vi "gui for machine parameters.vi"() -> ()   [LabVIEW 2025]
uses:
  control modification.ctl
  Control 5.ctl
  horizontal slide control.ctl
  counterweight load control.ctl
  time control.ctl
  <vilib>/picture/picture.llb/imagedata.ctl
  Control 6.ctl
  <vilib>/picture/picture.llb/Draw True-Color Pixmap.vi
panel:
  in  "stop 3":bool
  in  "dimension size":i32
  in  "Tank 3":T1 scale=0.0..100.0
  in  "Tank 2":T1 scale=0.0..100.0
  in  "Table 3":T2
  in  "?":bool
  in  "?":bool
  in  "?":bool
  in  "?":bool
  in  "?":bool
  in  "?":bool
  in  "?":bool
  in  "?":bool
  out "image data 2":T3
  in  "path to PNG file 2":path=path "C:/Dhanush/Dhanush/Vehicle articulated (1).PNG"
  in  "Rotation Angle (degree) 2":dbl(knob) scale=-180.0..180.0
  in  "Scale 2":dbl(slide)=1.0 scale=0.1..10.0
  in  "stop 2":bool
  out "?":picture
  out "?":T4
  out "?":T5 scale=0.0..6.0
  out "?":T5 scale=0.0..6.0
  out "image data":T3
  in  "path to PNG file":path=path "C:/Dhanush/Dhanush/Vehicle articulated (1).PNG"
  in  "Rotation Angle (degree)":dbl(knob) scale=-180.0..180.0
  in  "Scale":dbl(slide)=1.0 scale=0.1..10.0
  in  "stop":bool
  out "?":picture
  out "?":T4
  out "?":T6 scale=0.0..100.0
  in  "Table 2":T2
  in  "?":T7
  # "No of Cycles"
  # "Holding Time"
  # "Y axis Angle"
  # "Pressure"
  # "Automatic Mode Parameter Settings"
  # "Y axis"
  # "X axis"
  # "Cycle"
  # "Settings"
  # "%"
  # "Overall Progress Bar"
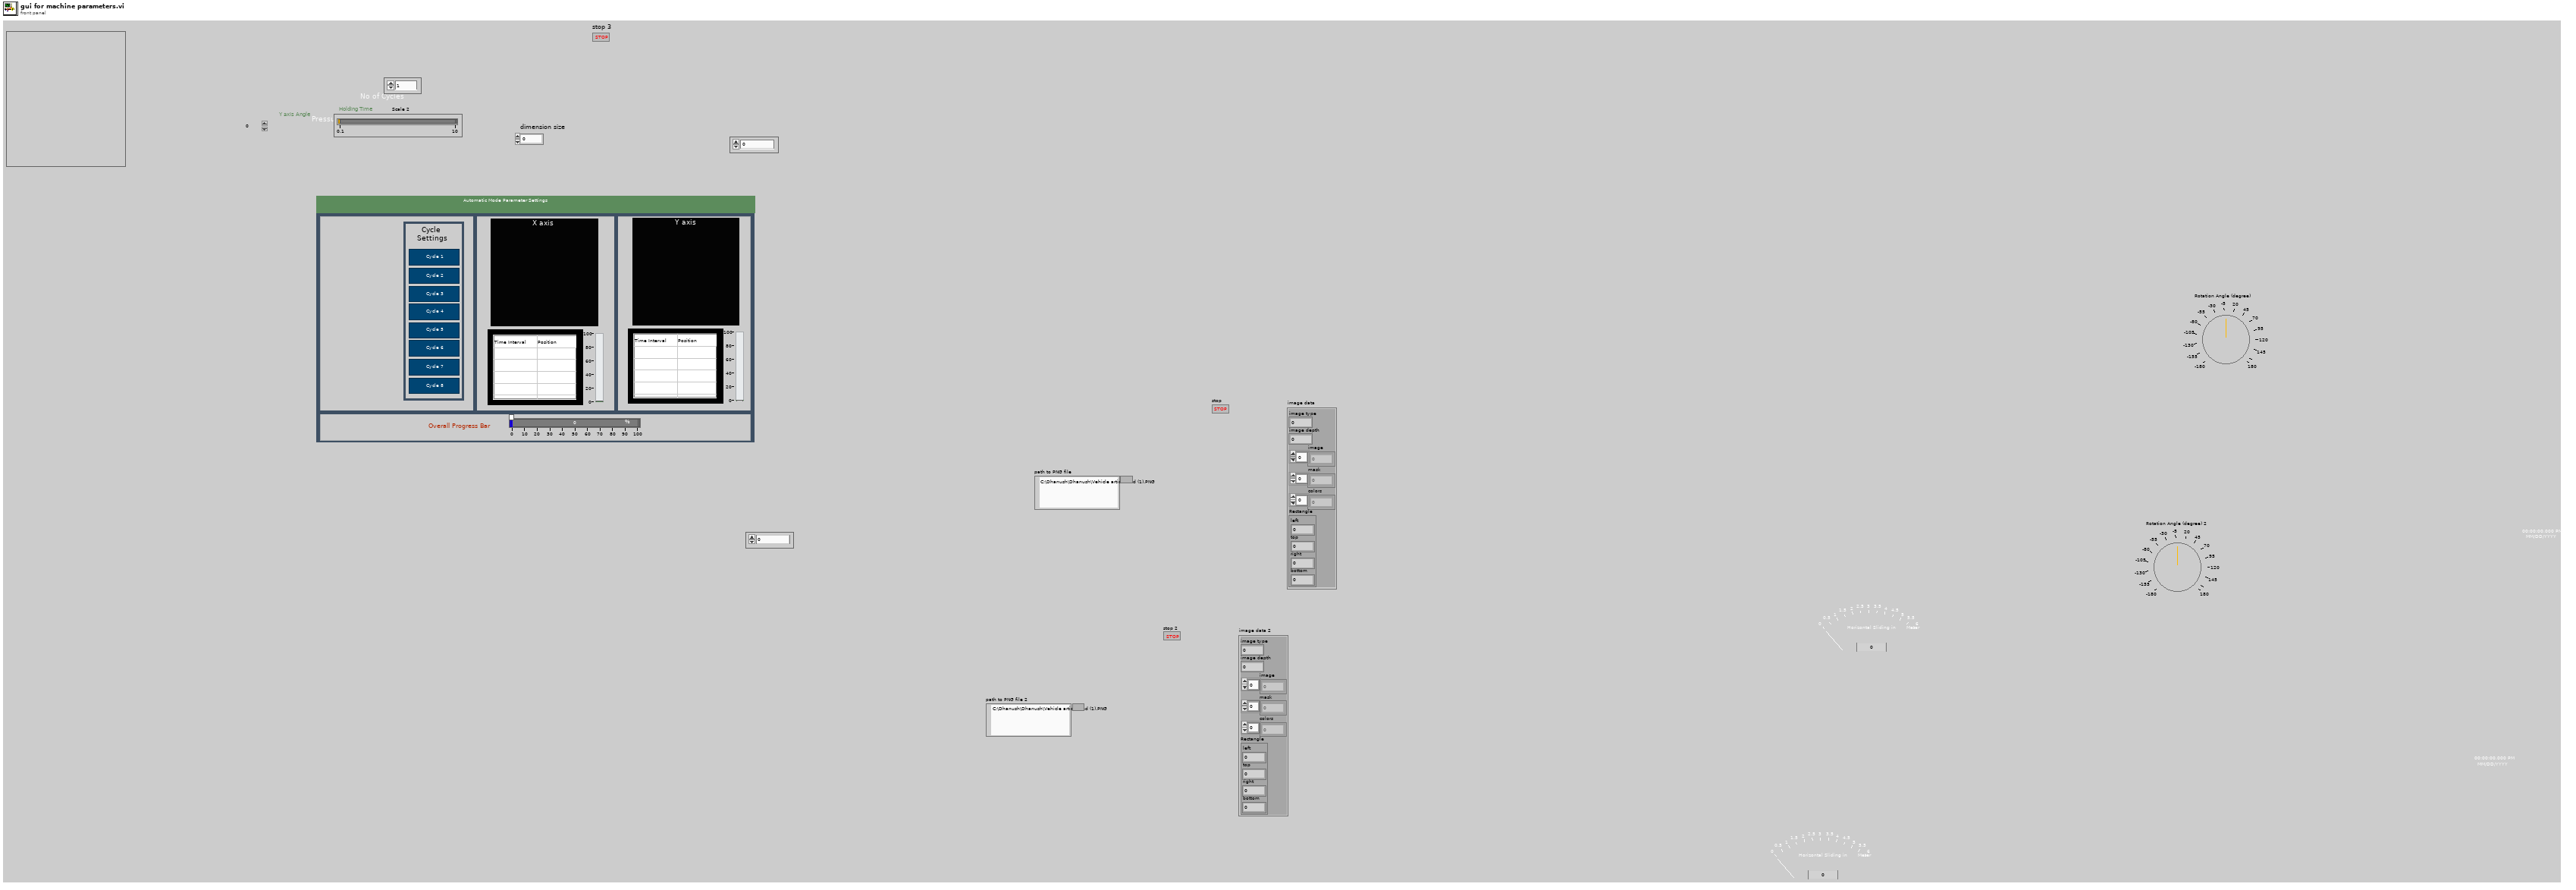
[diagram p1: front panel]
types:
  T1 = typedef "Control 6.ctl" = dbl
  T2 = typedef "Control 5.ctl" = string[][]
  T3 = typedef "imagedata.ctl" = cluster{"image type":i32, "image depth":i32, "image":u8[], "mask":u8[], "colors":u32[], "Rectangle":cluster{"left":i16, "top":i16, "right":i16, "bottom":i16}}
  T4 = typedef "time control.ctl" = timestamp
  T5 = typedef "counterweight load control.ctl" = dbl
  T6 = typedef "horizontal slide control.ctl" = dbl
  T7 = typedef "control modification.ctl" = dbl
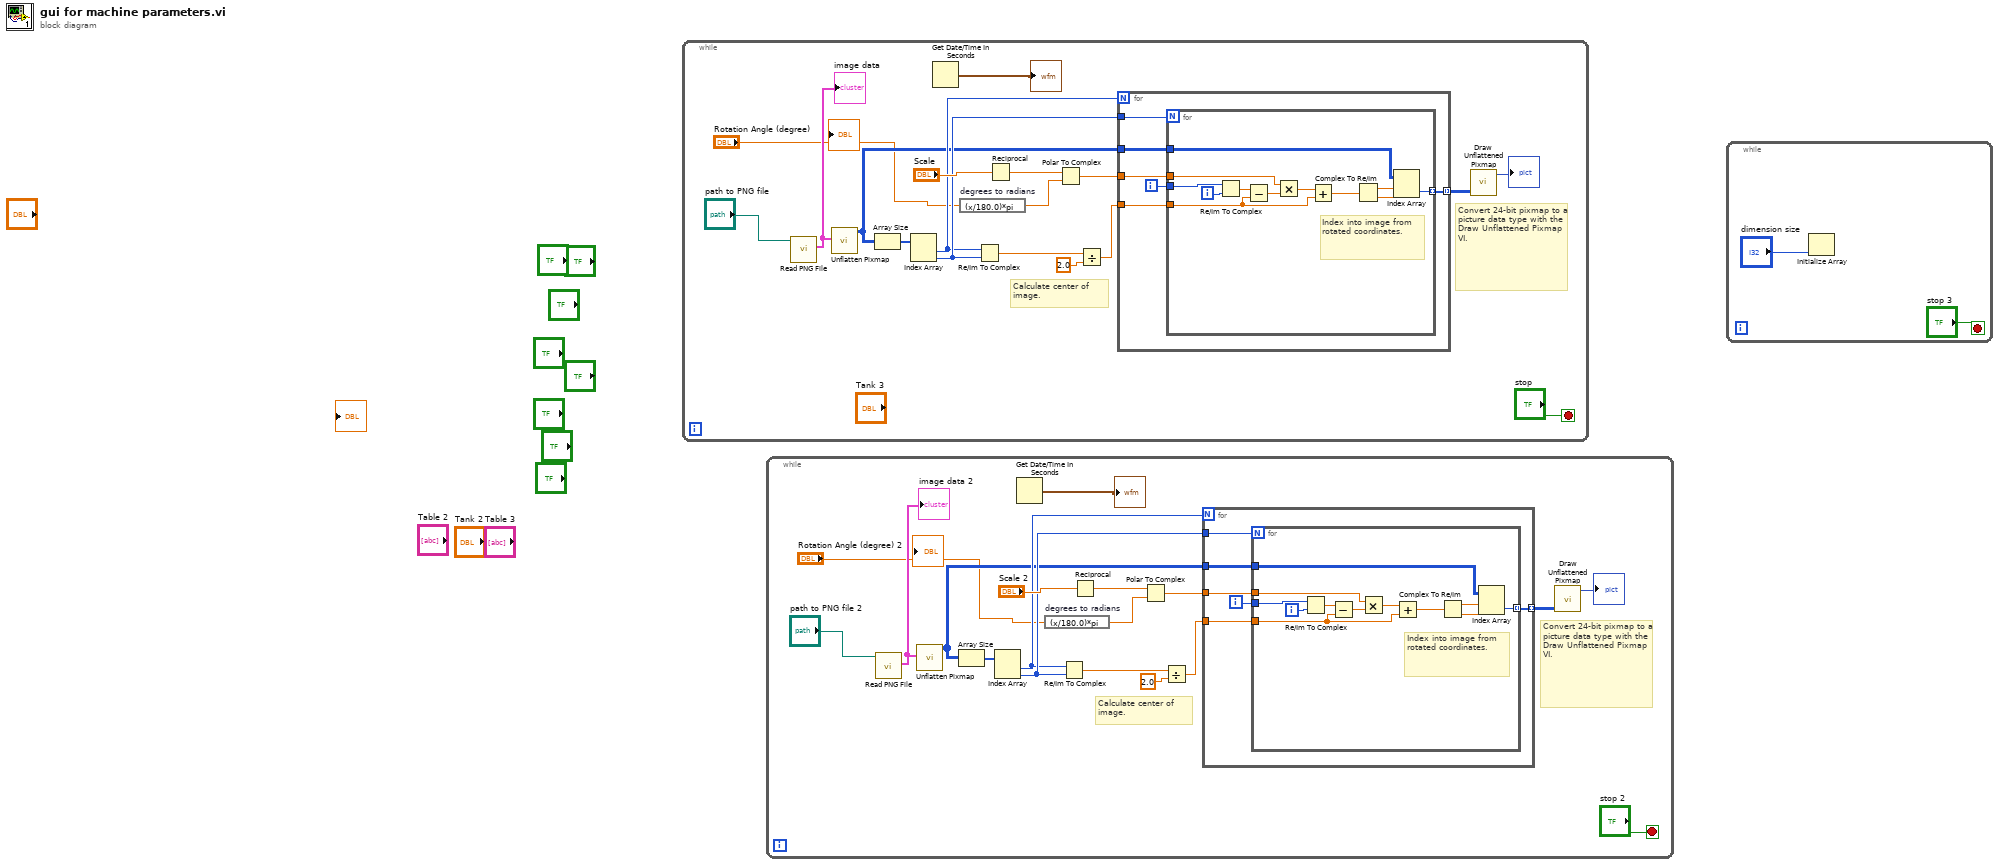
[diagram p0: block diagram]
diagram:
  n1 = while {
    stop <- "stop" stop-if-true
    # "Calculate center of image."
    # "Convert 24-bit pixmap to a picture data type with the Draw Unflattened Pixmap VI."
    n2 = call <vilib>:"Read PNG File.vi"("path to PNG file"="path to PNG file") -> ("image data"=w6:T3)  [unwired: 8 in, 2 out]
    "image data" <- w6
    n3 = call <vilib>:"Unflatten Pixmap.vi"("image data"=w6) -> ("24-bit pixmap"=w7:u32[][])  [unwired: 4 in, 6 out]
    n4 = Array Size(array=w7) -> (size(s)=w12:i32[])
    n5 = Index Array(array=w12) -> (element #1=w10:i32, element #2=w11:i32)  [unwired: 2 in]
    n6 = Get Date/Time In Seconds() -> (seconds since 1Jan1904=→"?":timestamp)
    n7 = expression code="(x/180.0)*pi" "degrees to radians"("Rotation Angle (degree)") -> (w5:dbl)
    n8 = Re/Im To Complex(1:w11, 2:w10) -> (0:w13:cdb)
    n9 = Reciprocal(x="Scale") -> (1/x=w15:dbl)
    n10 = Polar To Complex(1:w5, 2:w15) -> (0:w14:cdb)
    n11 = Divide(x=w13, y=2.0) -> (x/y=w9:cdb)
    n12 = for {
      N: w10 -> [_]
      tunnel: w11 -> [w23]
      tunnel: w7 -> [w22]
      tunnel: [w21] -> w17 mode=indexing
      tunnel: w14 -> [w20]
      tunnel: w9 -> [w19]
      i -> [w24]
      n13 = for {
        N: w23 -> [_]
        tunnel: w24 -> [w33]
        tunnel: w22 -> [w36]
        tunnel: [w35] -> w21 mode=indexing
        tunnel: w20 -> [w26]
        tunnel: w19 -> [w25]
        i -> [w34]
        # "Index into image from rotated coordinates."
        n14 = Re/Im To Complex(1:w34, 2:w33) -> (0:w32:cdb)
        n15 = Subtract(x=w32, y=w25) -> (x-y=w31:cdb)
        n16 = Multiply(x=w26, y=w31) -> (x*y=w30:cdb)
        n17 = Add(x=w30, y=w25) -> (x+y=w29:cdb)
        n18 = Complex To Re/Im(x + iy=w29) -> (x=w28:dbl, y=w27:dbl)
        n19 = Index Array(array=w36, index (row)=w28, index (col)=w27) -> (element=w35:u32)
      }
    }
    n20 = call-poly <vilib>:"Draw Unflattened Pixmap.vi"("data (RGB format)"=w17) -> ("new picture"=→"?":picture)  [unwired: 8 in]
  }
  n21 = while {
    stop <- "stop 2" stop-if-true
    # "Calculate center of image."
    # "Convert 24-bit pixmap to a picture data type with the Draw Unflattened Pixmap VI."
    n22 = call <vilib>:"Read PNG File.vi"("path to PNG file"="path to PNG file 2") -> ("image data"=w42:T3)  [unwired: 8 in, 2 out]
    "image data 2" <- w42
    n23 = call <vilib>:"Unflatten Pixmap.vi"("image data"=w42) -> ("24-bit pixmap"=w43:u32[][])  [unwired: 4 in, 6 out]
    n24 = Array Size(array=w43) -> (size(s)=w48:i32[])
    n25 = Index Array(array=w48) -> (element #1=w46:i32, element #2=w47:i32)  [unwired: 2 in]
    n26 = Get Date/Time In Seconds() -> (seconds since 1Jan1904=→"?":timestamp)
    n27 = expression code="(x/180.0)*pi" "degrees to radians"("Rotation Angle (degree) 2") -> (w41:dbl)
    n28 = Re/Im To Complex(1:w47, 2:w46) -> (0:w49:cdb)
    n29 = Reciprocal(x="Scale 2") -> (1/x=w51:dbl)
    n30 = Polar To Complex(1:w41, 2:w51) -> (0:w50:cdb)
    n31 = Divide(x=w49, y=2.0) -> (x/y=w45:cdb)
    n32 = for {
      N: w46 -> [_]
      tunnel: w47 -> [w59]
      tunnel: w43 -> [w58]
      tunnel: [w57] -> w53 mode=indexing
      tunnel: w50 -> [w56]
      tunnel: w45 -> [w55]
      i -> [w60]
      n33 = for {
        N: w59 -> [_]
        tunnel: w60 -> [w69]
        tunnel: w58 -> [w72]
        tunnel: [w71] -> w57 mode=indexing
        tunnel: w56 -> [w62]
        tunnel: w55 -> [w61]
        i -> [w70]
        # "Index into image from rotated coordinates."
        n34 = Re/Im To Complex(1:w70, 2:w69) -> (0:w68:cdb)
        n35 = Subtract(x=w68, y=w61) -> (x-y=w67:cdb)
        n36 = Multiply(x=w62, y=w67) -> (x*y=w66:cdb)
        n37 = Add(x=w66, y=w61) -> (x+y=w65:cdb)
        n38 = Complex To Re/Im(x + iy=w65) -> (x=w64:dbl, y=w63:dbl)
        n39 = Index Array(array=w72, index (row)=w64, index (col)=w63) -> (element=w71:u32)
      }
    }
    n40 = call-poly <vilib>:"Draw Unflattened Pixmap.vi"("data (RGB format)"=w53) -> ("new picture"=→"?":picture)  [unwired: 8 in]
  }
  n41 = while {
    stop <- "stop 3" stop-if-true
    n42 = Initialize Array("dimension size") -> ()  [unwired: 1 in, 1 out]
  }
